vi "Plugin Design Pattern.vi"   [LabVIEW 2011]
uses:
  Plugin Template/Generic Plugin.lvclass
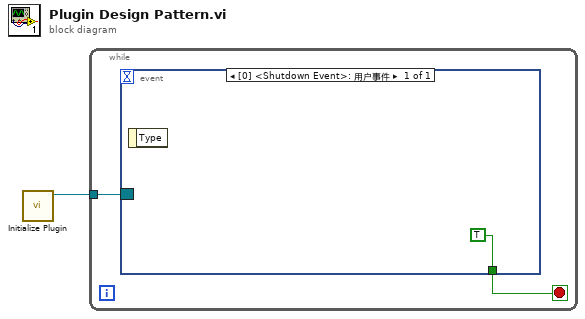
[diagram p0: block diagram]
diagram:
  n1 = call "Initialize Plugin.vi"() -> ("Event Registration Refnum"=w1:refnum<event-registration>)  [unwired: 9 in, 2 out]
  n2 = while {
    tunnel: w1 -> [w3]
    stop <- w2 stop-if-true
    n3 = event shown="[0] <Shutdown Event>: 用户事件" {
      selector: w3 -> [_]
      dyn-events: _ -> [_]
      timeout: _ -> [_]
      tunnel: [TRUE] -> w2
      event User Event {
        n4 = event-data() -> ()  [unwired: 1 in, 1 out]
      }
    }
  }
